vi "draw.vi"(8 "error in (no error)":errorcluster, 11 "Parcour_element in":refnum<class "Parcour_element.lvclass">) -> (0 "error out":errorcluster, 2 "element":cluster{"x":dbl[], "y":dbl[]}, 3 "Parcour_element out":refnum<class "Parcour_element.lvclass">)   [LabVIEW 2019, in "Parcour_element.lvclass"]
uses:
  Parcour_element.lvclass
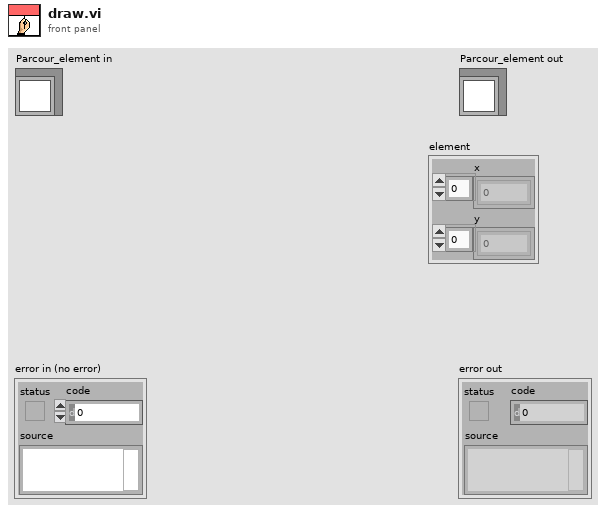
[diagram p1: front panel]
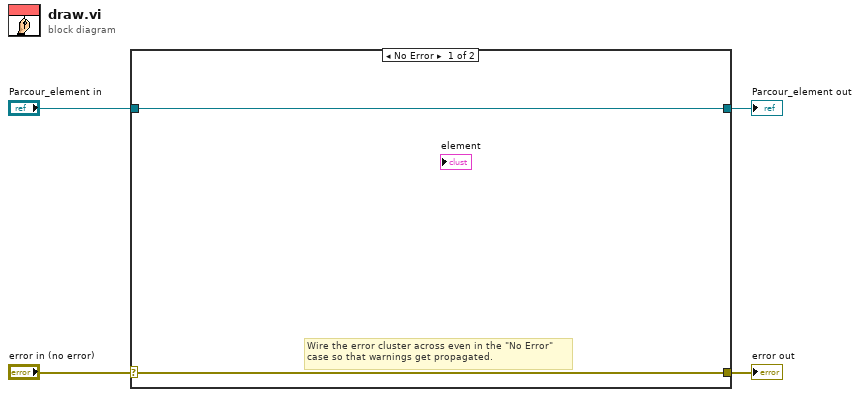
[diagram p0: block diagram]
diagram:
  n1 = case shown="No Error" "error in (no error)" {
    selector: "error in (no error)" -> [w5 w8]
    tunnel: [w5 w8] -> w3
    tunnel: [w6 w7] -> w1
    tunnel: "Parcour_element in" -> [w6 w7]
    frame No Error {
      # "Wire the error cluster across even in the \"No Error\"\ncase so that warnings get propagated."
    }
    frame Error {
    }
  }
  "error out" <- w3
  "Parcour_element out" <- w1
